vi "Lecture 3 - Finite State Machine.vi"() -> ()   [LabVIEW 2019]
panel:
  out "My Counter":i32
  in  "stop":bool
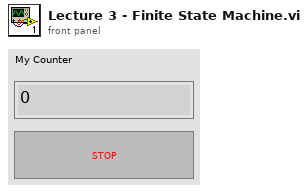
[diagram p1: front panel]
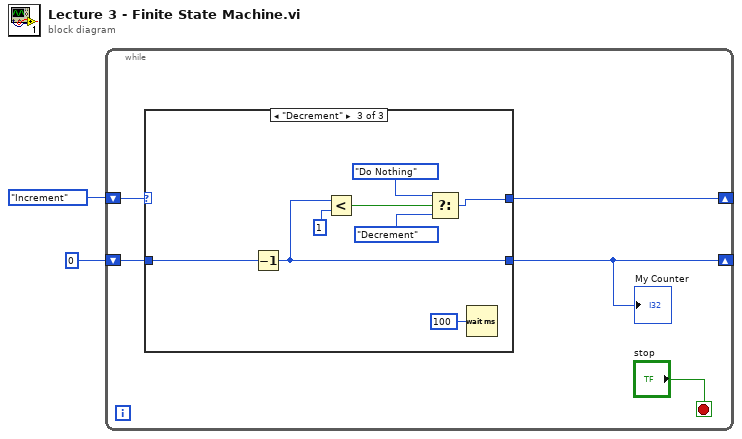
[diagram p0: block diagram]
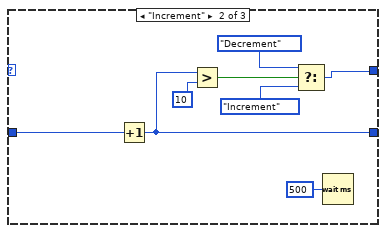
[diagram p3: hidden frame]
diagram:
  n1 = while {
    shift-right: [w5] -> _
    shift-left: enum16{"Do Nothing", "Increment", "Decrement"}."Increment" -> [w6]
    shift-right: [w3] -> _
    shift-left: 0 -> [w4]
    stop <- "stop" stop-if-true
    n2 = case shown="\"Decrement\"" w6 {
      selector: w6 -> [w9 _ _]
      tunnel: [w9 w11 w19] -> w5
      tunnel: w4 -> [w8 w17 w25]
      tunnel: [w8 w14 w20] -> w3
      frame "Do Nothing", Default {
      }
      frame "Increment" {
        n3 = Increment(x=w17) -> (x+1=w14:i32)
        n4 = Greater?(x=w14, y=10) -> (0:w15:bool)
        n5 = Select(t=enum16{"Do Nothing", "Increment", "Decrement"}."Decrement", s=w15, f=enum16{"Do Nothing", "Increment", "Decrement"}."Increment") -> (s? t:f=w11:enum16{"Do Nothing", "Increment", "Decrement"})
        n6 = Wait (ms)(milliseconds to wait=u32 500) -> ()  [unwired: 1 out]
      }
      frame "Decrement" {
        n7 = Decrement(x=w25) -> (x-1=w20:i32)
        n8 = Less?(x=w20, y=1) -> (x < y?=w23:bool)
        n9 = Select(t=enum16{"Do Nothing", "Increment", "Decrement"}."Do Nothing", s=w23, f=enum16{"Do Nothing", "Increment", "Decrement"}."Decrement") -> (s? t:f=w19:enum16{"Do Nothing", "Increment", "Decrement"})
        n10 = Wait (ms)(milliseconds to wait=u32 100) -> ()  [unwired: 1 out]
      }
    }
    "My Counter" <- w3
  }
